vi "glueing_proc.vi"() -> ()   [LabVIEW 2011]
panel:
  in  "fine tuning y \nmove +2 mm":bool
  in  "fine tuning x \nmove - 2 mm":bool
  in  "fine tuning y \nmove - 2 mm":bool
  in  "fine tuning x \nmove + 2 mm":bool
  in  "discharge glue":bool
  in  "Start 2":bool
  in  "spint down - II part":bool
  in  "glue press 2mm - II part":bool
  in  "spint down - II part":bool
  in  "zero done 2":bool
  in  "zero Gluer - end":bool
  in  "zero x - end":bool
  in  "zero y - end":bool
  in  "zero Spint - end":bool
  in  "zero Spint for replacing glue":bool
  in  "spint down 2":bool
  in  "glue press 2mm":bool
  in  "spint down":bool
  in  "Start":bool
  in  "fine tuning z dw 1mm":bool
  in  "fine tuning z up 1mm":bool
  in  "goto z pos 2":bool
  in  "goto z pos":bool
  in  "goto y pos":bool
  in  "positioning done":bool
  in  "goto x pos":bool
  in  "zero Spint":bool
  out "output":string
  out "command":string
  in  "zero done":bool
  in  "zero Gluer":bool
  in  "zero x":bool
  in  "zero y":bool
  # "Posiziono in zero"
  # "Vado in posizione"
  # "Fine tuning in posizione x e y \nsolo se necessario"
  # "Muovo spintore e inizio a incollare"
  # "Cambio cartuccia della colla\n\nSTART riprende incollaggio"
  # "Scarico la colla e \nritorno a zero"
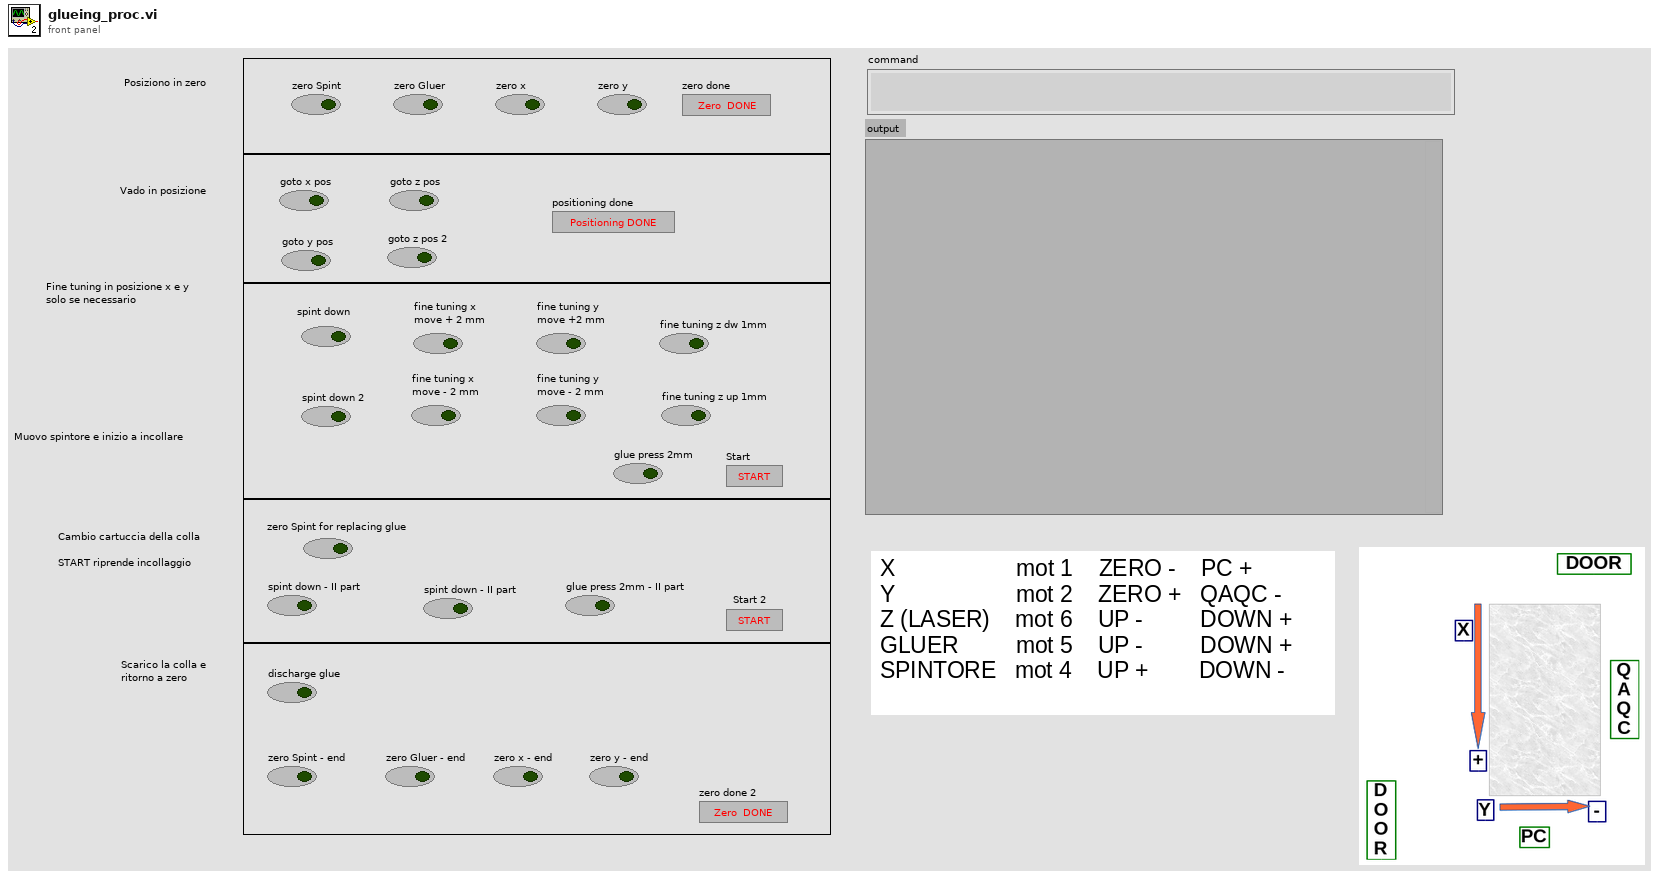
[diagram p1: front panel]
types:
  T1 = enum16{"open", "replace", "create", "open or create", "replace or create", "replace or create with confirmation"}
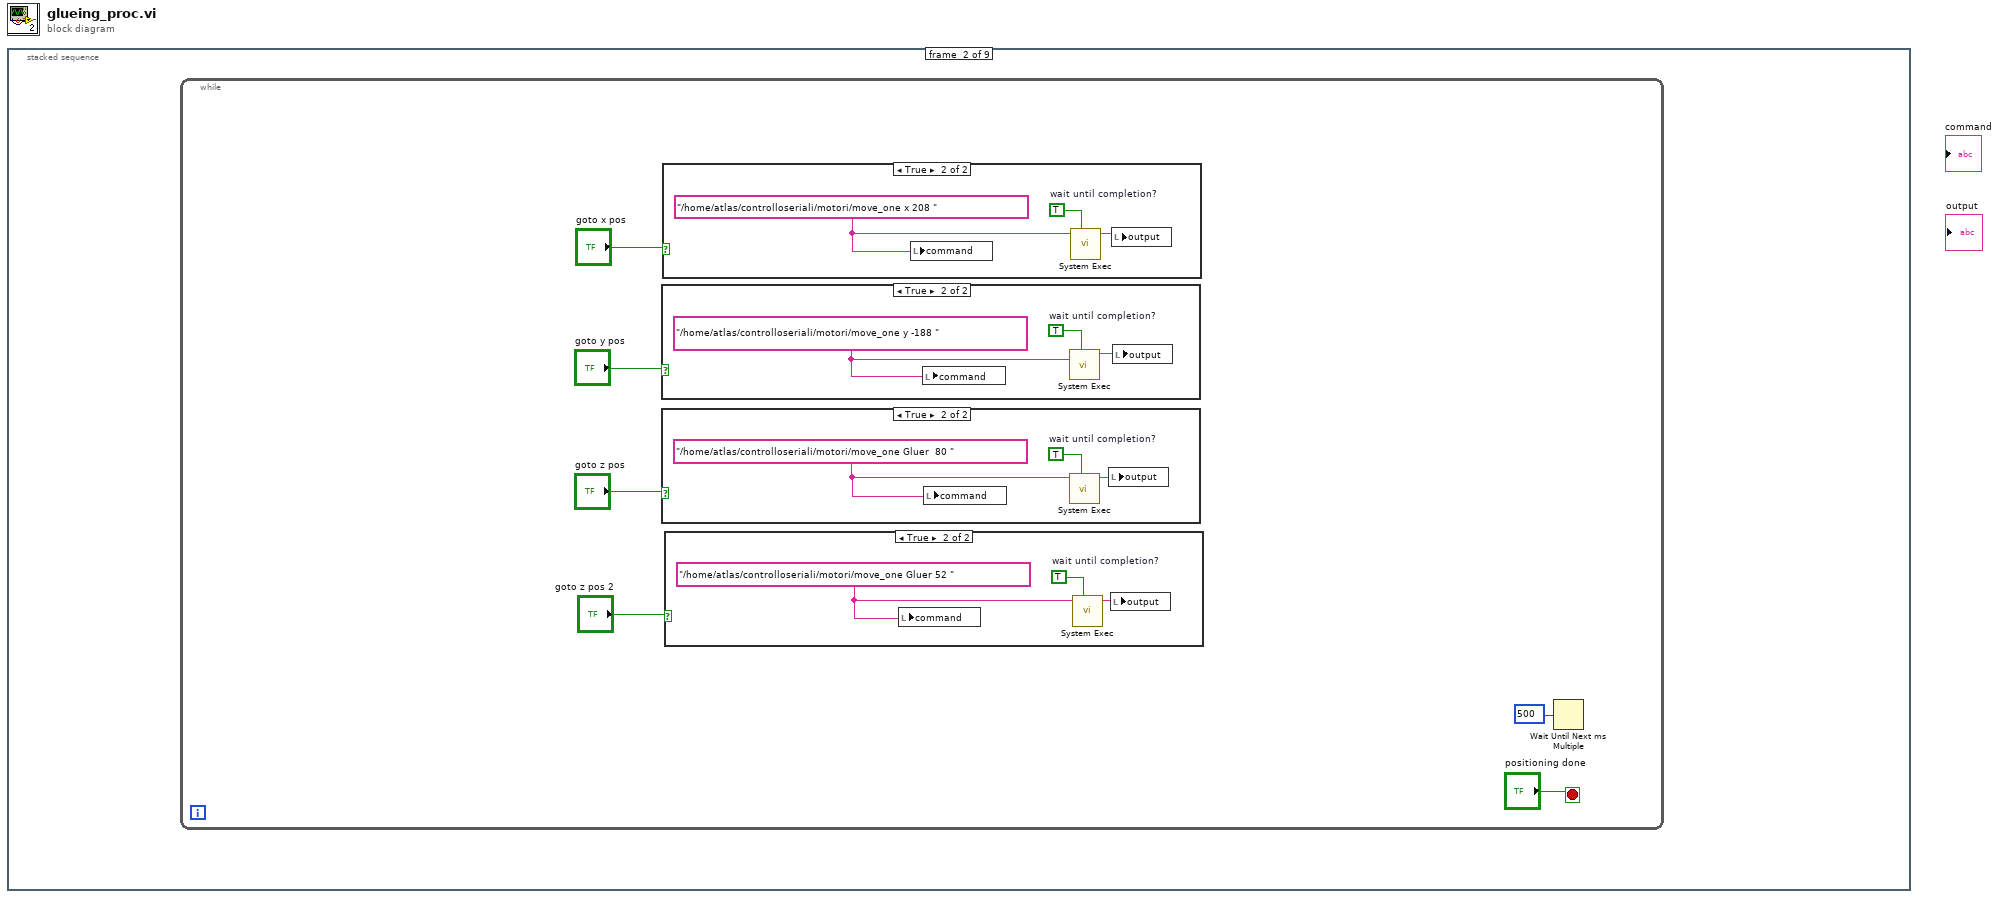
[diagram p0: block diagram]
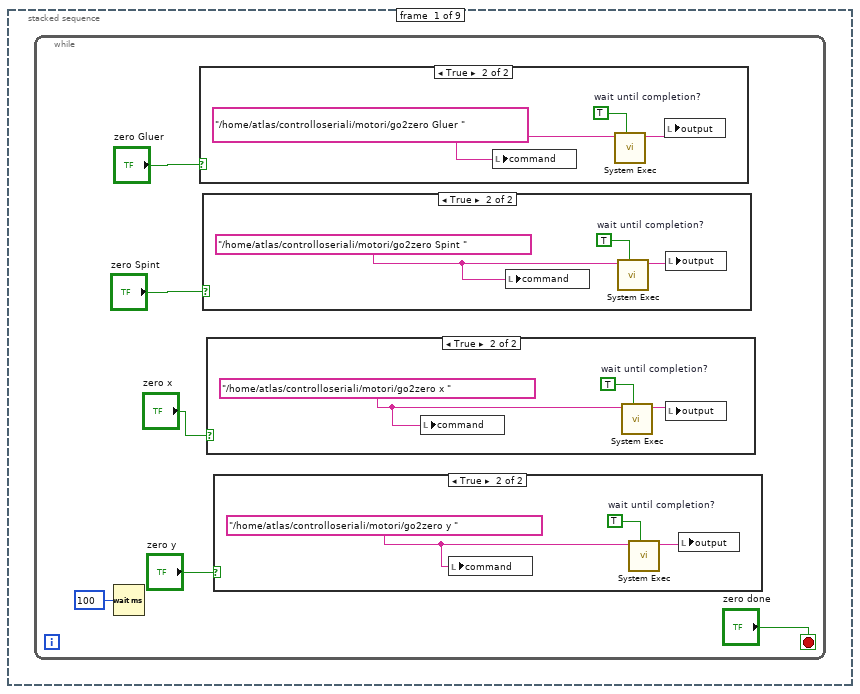
[diagram p2: hidden frame]
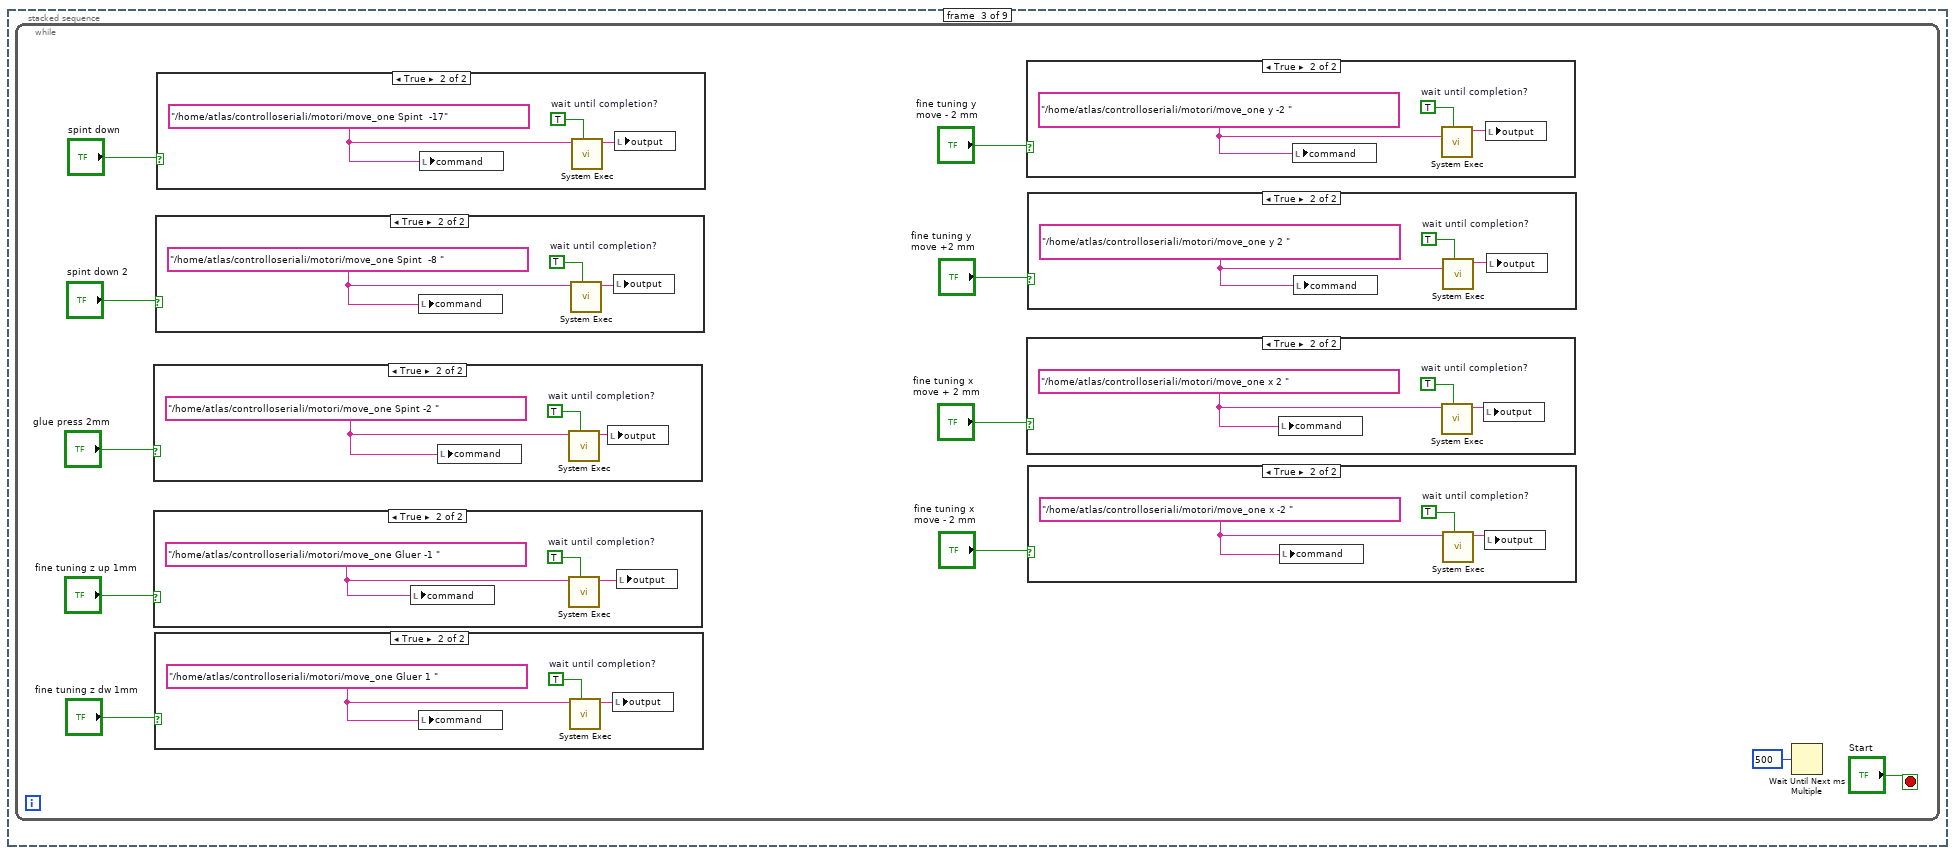
[diagram p11: hidden frame]
diagram:
  n1 = stacked-sequence {
    frame #0 {
      n2 = while {
        stop <- "zero done" stop-if-true
        n3 = Wait (ms)(milliseconds to wait=u32 100) -> ()  [unwired: 1 out]
        n4 = case shown="True" "zero Gluer" {
          frame False {
          }
          frame True {
            w17 = "/home/atlas/controlloseriali/motori/go2zero Gluer " ("string")
            w18 = TRUE  # wait until completion?
            n5 = local write "command"(w17) -> ()
            n6 = call <vilib>:"System Exec.vi"("wait until completion? (T)"=w18, "command line"=w17) -> ("standard output"=w16:string)  [unwired: 6 in, 3 out]
            n7 = local write "output"(w16) -> ()
          }
        }
        n8 = case shown="True" "zero Spint" {
          frame False {
          }
          frame True {
            w7 = "/home/atlas/controlloseriali/motori/go2zero Spint " ("string")
            w9 = TRUE  # wait until completion?
            n9 = local write "command"(w7) -> ()
            n10 = call <vilib>:"System Exec.vi"("wait until completion? (T)"=w9, "command line"=w7) -> ("standard output"=w8:string)  [unwired: 6 in, 3 out]
            n11 = local write "output"(w8) -> ()
          }
        }
        n12 = case shown="True" "zero x" {
          frame False {
          }
          frame True {
            w14 = "/home/atlas/controlloseriali/motori/go2zero x " ("string")
            w15 = TRUE  # wait until completion?
            n13 = local write "command"(w14) -> ()
            n14 = call <vilib>:"System Exec.vi"("wait until completion? (T)"=w15, "command line"=w14) -> ("standard output"=w13:string)  [unwired: 6 in, 3 out]
            n15 = local write "output"(w13) -> ()
          }
        }
        n16 = case shown="True" "zero y" {
          frame False {
          }
          frame True {
            w11 = "/home/atlas/controlloseriali/motori/go2zero y " ("string")
            w12 = TRUE  # wait until completion?
            n17 = local write "command"(w11) -> ()
            n18 = call <vilib>:"System Exec.vi"("wait until completion? (T)"=w12, "command line"=w11) -> ("standard output"=w10:string)  [unwired: 6 in, 3 out]
            n19 = local write "output"(w10) -> ()
          }
        }
      }
    }
    frame #1 {
      n20 = while {
        stop <- "positioning done" stop-if-true
        n21 = case shown="True" "goto y pos" {
          frame False {
          }
          frame True {
            w31 = "/home/atlas/controlloseriali/motori/move_one y -188 " ("string")
            w33 = TRUE  # wait until completion?
            n22 = local write "command"(w31) -> ()
            n23 = call <vilib>:"System Exec.vi"("wait until completion? (T)"=w33, "command line"=w31) -> ("standard output"=w32:string)  [unwired: 6 in, 3 out]
            n24 = local write "output"(w32) -> ()
          }
        }
        n25 = case shown="True" "goto z pos" {
          frame False {
          }
          frame True {
            w28 = "/home/atlas/controlloseriali/motori/move_one Gluer  80 " ("string")
            w30 = TRUE  # wait until completion?
            n26 = local write "command"(w28) -> ()
            n27 = call <vilib>:"System Exec.vi"("wait until completion? (T)"=w30, "command line"=w28) -> ("standard output"=w29:string)  [unwired: 6 in, 3 out]
            n28 = local write "output"(w29) -> ()
          }
        }
        n29 = case shown="True" "goto x pos" {
          frame False {
          }
          frame True {
            w34 = "/home/atlas/controlloseriali/motori/move_one x 208 " ("string")
            w36 = TRUE  # wait until completion?
            n30 = local write "command"(w34) -> ()
            n31 = call <vilib>:"System Exec.vi"("wait until completion? (T)"=w36, "command line"=w34) -> ("standard output"=w35:string)  [unwired: 6 in, 3 out]
            n32 = local write "output"(w35) -> ()
          }
        }
        n33 = case shown="True" "goto z pos 2" {
          frame False {
          }
          frame True {
            w25 = "/home/atlas/controlloseriali/motori/move_one Gluer 52 " ("string")
            w27 = TRUE  # wait until completion?
            n34 = local write "command"(w25) -> ()
            n35 = call <vilib>:"System Exec.vi"("wait until completion? (T)"=w27, "command line"=w25) -> ("standard output"=w26:string)  [unwired: 6 in, 3 out]
            n36 = local write "output"(w26) -> ()
          }
        }
        n37 = Wait Until Next ms Multiple(millisecond multiple=u32 500) -> ()  [unwired: 1 out]
      }
    }
    frame #2 {
      n38 = while {
        stop <- "Start" stop-if-true
        n39 = case shown="True" "glue press 2mm" {
          frame False {
          }
          frame True {
            w70 = "/home/atlas/controlloseriali/motori/move_one Spint -2 " ("string")
            w71 = TRUE  # wait until completion?
            n40 = local write "command"(w70) -> ()
            n41 = call <vilib>:"System Exec.vi"("wait until completion? (T)"=w71, "command line"=w70) -> ("standard output"=w69:string)  [unwired: 6 in, 3 out]
            n42 = local write "output"(w69) -> ()
          }
        }
        n43 = case shown="True" "fine tuning z up 1mm" {
          frame False {
          }
          frame True {
            w51 = "/home/atlas/controlloseriali/motori/move_one Gluer -1 " ("string")
            w53 = TRUE  # wait until completion?
            n44 = local write "command"(w51) -> ()
            n45 = call <vilib>:"System Exec.vi"("wait until completion? (T)"=w53, "command line"=w51) -> ("standard output"=w52:string)  [unwired: 6 in, 3 out]
            n46 = local write "output"(w52) -> ()
          }
        }
        n47 = case shown="True" "fine tuning z dw 1mm" {
          frame False {
          }
          frame True {
            w48 = "/home/atlas/controlloseriali/motori/move_one Gluer 1 " ("string")
            w50 = TRUE  # wait until completion?
            n48 = local write "command"(w48) -> ()
            n49 = call <vilib>:"System Exec.vi"("wait until completion? (T)"=w50, "command line"=w48) -> ("standard output"=w49:string)  [unwired: 6 in, 3 out]
            n50 = local write "output"(w49) -> ()
          }
        }
        n51 = case shown="True" "spint down 2" {
          frame False {
          }
          frame True {
            w66 = "/home/atlas/controlloseriali/motori/move_one Spint  -8 " ("string")
            w68 = TRUE  # wait until completion?
            n52 = local write "command"(w66) -> ()
            n53 = call <vilib>:"System Exec.vi"("wait until completion? (T)"=w68, "command line"=w66) -> ("standard output"=w67:string)  [unwired: 6 in, 3 out]
            n54 = local write "output"(w67) -> ()
          }
        }
        n55 = case shown="True" "spint down" {
          frame False {
          }
          frame True {
            w72 = "/home/atlas/controlloseriali/motori/move_one Spint  -17" ("string")
            w74 = TRUE  # wait until completion?
            n56 = local write "command"(w72) -> ()
            n57 = call <vilib>:"System Exec.vi"("wait until completion? (T)"=w74, "command line"=w72) -> ("standard output"=w73:string)  [unwired: 6 in, 3 out]
            n58 = local write "output"(w73) -> ()
          }
        }
        n59 = case shown="True" "fine tuning y \nmove - 2 mm" {
          frame False {
          }
          frame True {
            w63 = "/home/atlas/controlloseriali/motori/move_one y -2 " ("string")
            w65 = TRUE  # wait until completion?
            n60 = local write "command"(w63) -> ()
            n61 = call <vilib>:"System Exec.vi"("wait until completion? (T)"=w65, "command line"=w63) -> ("standard output"=w64:string)  [unwired: 6 in, 3 out]
            n62 = local write "output"(w64) -> ()
          }
        }
        n63 = case shown="True" "fine tuning x \nmove + 2 mm" {
          frame False {
          }
          frame True {
            w57 = "/home/atlas/controlloseriali/motori/move_one x 2 " ("string")
            w59 = TRUE  # wait until completion?
            n64 = local write "command"(w57) -> ()
            n65 = call <vilib>:"System Exec.vi"("wait until completion? (T)"=w59, "command line"=w57) -> ("standard output"=w58:string)  [unwired: 6 in, 3 out]
            n66 = local write "output"(w58) -> ()
          }
        }
        n67 = case shown="True" "fine tuning y \nmove +2 mm" {
          frame False {
          }
          frame True {
            w60 = "/home/atlas/controlloseriali/motori/move_one y 2 " ("string")
            w62 = TRUE  # wait until completion?
            n68 = local write "command"(w60) -> ()
            n69 = call <vilib>:"System Exec.vi"("wait until completion? (T)"=w62, "command line"=w60) -> ("standard output"=w61:string)  [unwired: 6 in, 3 out]
            n70 = local write "output"(w61) -> ()
          }
        }
        n71 = case shown="True" "fine tuning x \nmove - 2 mm" {
          frame False {
          }
          frame True {
            w54 = "/home/atlas/controlloseriali/motori/move_one x -2 " ("string")
            w56 = TRUE  # wait until completion?
            n72 = local write "command"(w54) -> ()
            n73 = call <vilib>:"System Exec.vi"("wait until completion? (T)"=w56, "command line"=w54) -> ("standard output"=w55:string)  [unwired: 6 in, 3 out]
            n74 = local write "output"(w55) -> ()
          }
        }
        n75 = Wait Until Next ms Multiple(millisecond multiple=u32 500) -> ()  [unwired: 1 out]
      }
    }
    frame #3 {
      n76 = flat-sequence {
        frame #0 {
          n77 = Open/Create/Replace File(file path (use dialog)=path "/tmp/glueing.tmp", operation (0:open)=T1."open or create") -> ()  [unwired: 4 in, 3 out]
          n78 = call <vilib>:"System Exec.vi"("wait until completion? (T)"=FALSE, "command line"="gnome-terminal -e \"tail -f /tmp/glueing.tmp\"" ("logwindow")) -> ()  [unwired: 6 in, 4 out]
        }
        frame #1 {
          w85 = TRUE  # wait until completion?
          # "parametri ottimizzati per incollaggio"
          n79 = Concatenate Strings("/home/atlas/controlloseriali/fieldpoint/trap_XYS  " ("string"), "" ("string"), "-n 25 -x 33 60 -y  -1218 20 -s -4.1 17 " ("string"), "  | tee /tmp/glueing.tmp" ("string")) -> (w80:string)
          n80 = local write "command"(w80) -> ()
          n81 = call <vilib>:"System Exec.vi"("wait until completion? (T)"=w85, "command line"=w80) -> ("standard output"=w79:string)  [unwired: 6 in, 3 out]
          n82 = local write "output"(w79) -> ()
        }
      }
    }
    frame #4 {
      n83 = while {
        stop <- w87 stop-if-true
        n84 = case shown="True" "zero Spint for replacing glue" {
          tunnel: [FALSE TRUE] -> w87
          frame False {
          }
          frame True {
            w91 = "/home/atlas/controlloseriali/motori/go2zero Spint " ("string")
            w93 = TRUE  # wait until completion?
            n85 = local write "command"(w91) -> ()
            n86 = call <vilib>:"System Exec.vi"("wait until completion? (T)"=w93, "command line"=w91) -> ("standard output"=w92:string)  [unwired: 6 in, 3 out]
            n87 = local write "output"(w92) -> ()
          }
        }
        n88 = Wait (ms)(milliseconds to wait=u32 100) -> ()  [unwired: 1 out]
      }
    }
    frame #5 {
      n89 = One Button Dialog(message="Replace the glue!\nPress OK after done") -> ()  [unwired: 1 in, 1 out]
    }
    frame #6 {
      n90 = while {
        stop <- "Start 2" stop-if-true
        n91 = case shown="True" "glue press 2mm - II part" {
          frame False {
          }
          frame True {
            w104 = "/home/atlas/controlloseriali/motori/move_one Spint -2 " ("string")
            w105 = TRUE  # wait until completion?
            n92 = local write "command"(w104) -> ()
            n93 = call <vilib>:"System Exec.vi"("wait until completion? (T)"=w105, "command line"=w104) -> ("standard output"=w103:string)  [unwired: 6 in, 3 out]
            n94 = local write "output"(w103) -> ()
          }
        }
        n95 = case shown="True" "spint down - II part" {
          frame False {
          }
          frame True {
            w100 = "/home/atlas/controlloseriali/motori/move_one Spint  -8 " ("string")
            w102 = TRUE  # wait until completion?
            n96 = local write "command"(w100) -> ()
            n97 = call <vilib>:"System Exec.vi"("wait until completion? (T)"=w102, "command line"=w100) -> ("standard output"=w101:string)  [unwired: 6 in, 3 out]
            n98 = local write "output"(w101) -> ()
          }
        }
        n99 = case shown="True" "spint down - II part" {
          frame False {
          }
          frame True {
            w106 = "/home/atlas/controlloseriali/motori/move_one Spint  -17" ("string")
            w108 = TRUE  # wait until completion?
            n100 = local write "command"(w106) -> ()
            n101 = call <vilib>:"System Exec.vi"("wait until completion? (T)"=w108, "command line"=w106) -> ("standard output"=w107:string)  [unwired: 6 in, 3 out]
            n102 = local write "output"(w107) -> ()
          }
        }
        n103 = Wait Until Next ms Multiple(millisecond multiple=u32 500) -> ()  [unwired: 1 out]
      }
    }
    frame #7 {
      n104 = flat-sequence {
        frame #0 {
          n105 = Open/Create/Replace File(file path (use dialog)=path "/tmp/glueing.tmp", operation (0:open)=T1."open or create") -> ()  [unwired: 4 in, 3 out]
          n106 = call <vilib>:"System Exec.vi"("wait until completion? (T)"=FALSE, "command line"="gnome-terminal -e \"tail -f /tmp/glueing.tmp\"" ("logwindow")) -> ()  [unwired: 6 in, 4 out]
        }
        frame #1 {
          w119 = TRUE  # wait until completion?
          # "parametri ottimizzati per incollaggio"
          n107 = Concatenate Strings("/home/atlas/controlloseriali/fieldpoint/trap_XYS  " ("string"), "" ("string"), "-n 42 -x 33 60 -y  904 20 -s -3.1 17 " ("string"), "  | tee /tmp/glueing.tmp" ("string")) -> (w114:string)
          n108 = local write "command"(w114) -> ()
          n109 = call <vilib>:"System Exec.vi"("wait until completion? (T)"=w119, "command line"=w114) -> ("standard output"=w113:string)  [unwired: 6 in, 3 out]
          n110 = local write "output"(w113) -> ()
        }
      }
    }
    frame #8 {
      n111 = while {
        stop <- "zero done 2" stop-if-true
        n112 = Wait (ms)(milliseconds to wait=u32 100) -> ()  [unwired: 1 out]
        n113 = case shown="True" "discharge glue" {
          frame False {
          }
          frame True {
            w128 = "/home/atlas/controlloseriali/motori/move_one Spint  10 " ("string")
            w129 = TRUE  # wait until completion?
            n114 = local write "command"(w128) -> ()
            n115 = call <vilib>:"System Exec.vi"("wait until completion? (T)"=w129, "command line"=w128) -> ("standard output"=w127:string)  [unwired: 6 in, 3 out]
            n116 = local write "output"(w127) -> ()
          }
        }
        n117 = case shown="True" "zero Gluer - end" {
          frame False {
          }
          frame True {
            w140 = "/home/atlas/controlloseriali/motori/go2zero Gluer " ("string")
            w141 = TRUE  # wait until completion?
            n118 = local write "command"(w140) -> ()
            n119 = call <vilib>:"System Exec.vi"("wait until completion? (T)"=w141, "command line"=w140) -> ("standard output"=w139:string)  [unwired: 6 in, 3 out]
            n120 = local write "output"(w139) -> ()
          }
        }
        n121 = case shown="True" "zero Spint - end" {
          frame False {
          }
          frame True {
            w130 = "/home/atlas/controlloseriali/motori/go2zero Spint " ("string")
            w132 = TRUE  # wait until completion?
            n122 = local write "command"(w130) -> ()
            n123 = call <vilib>:"System Exec.vi"("wait until completion? (T)"=w132, "command line"=w130) -> ("standard output"=w131:string)  [unwired: 6 in, 3 out]
            n124 = local write "output"(w131) -> ()
          }
        }
        n125 = case shown="True" "zero x - end" {
          frame False {
          }
          frame True {
            w137 = "/home/atlas/controlloseriali/motori/go2zero x " ("string")
            w138 = TRUE  # wait until completion?
            n126 = local write "command"(w137) -> ()
            n127 = call <vilib>:"System Exec.vi"("wait until completion? (T)"=w138, "command line"=w137) -> ("standard output"=w136:string)  [unwired: 6 in, 3 out]
            n128 = local write "output"(w136) -> ()
          }
        }
        n129 = case shown="True" "zero y - end" {
          frame False {
          }
          frame True {
            w134 = "/home/atlas/controlloseriali/motori/go2zero y " ("string")
            w135 = TRUE  # wait until completion?
            n130 = local write "command"(w134) -> ()
            n131 = call <vilib>:"System Exec.vi"("wait until completion? (T)"=w135, "command line"=w134) -> ("standard output"=w133:string)  [unwired: 6 in, 3 out]
            n132 = local write "output"(w133) -> ()
          }
        }
      }
    }
  }
